vi "mini-proj.vi"() -> ()   [LabVIEW 2013]
uses:
  <vilib>/DAQmx/read.llb/DAQmx Read (Analog 1D Wfm NChan NSamp).vi
  <vilib>/DAQmx/miscellaneous.llb/DAQmx Fill In Error Info.vi
panel:
  out "rpm":dbl
  out "Graphe":waveform(dbl)[](graph)
  in  "Nom de tâche DAQmx":refnum<k21>
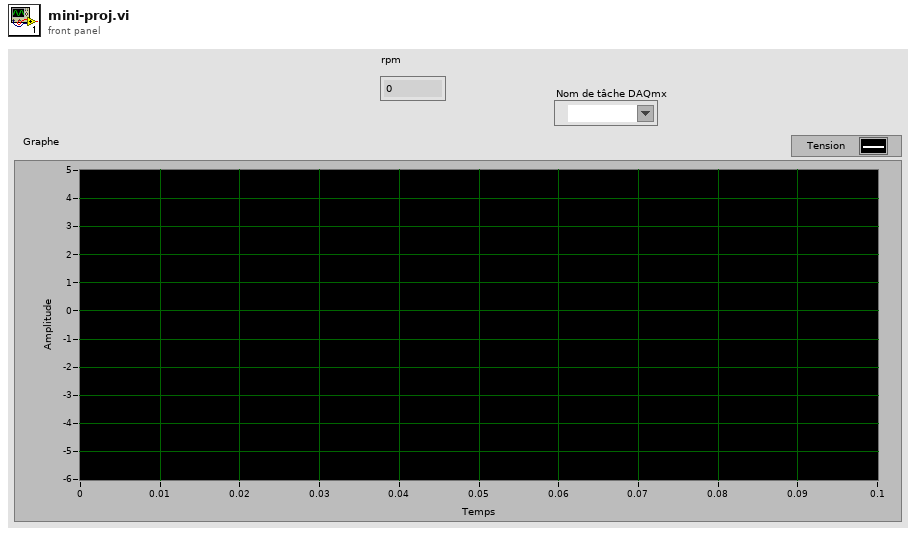
[diagram p1: front panel]
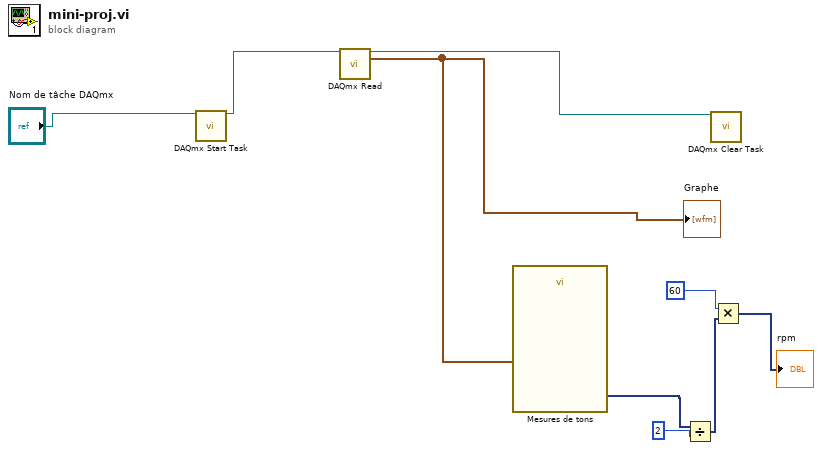
[diagram p0: block diagram]
diagram:
  n1 = call <vilib>:"DAQmx Start Task.vi"("task/channels in"="Nom de tâche DAQmx") -> ("task out"=w7:refnum<k21>)  [unwired: 13 in, 1 out]
  n2 = call-poly <vilib>:"DAQmx Read.vi"("task/channels in"=w7) -> ("task out"=w8:refnum<k21>, "data"=w6:waveform(dbl)[])  [unwired: 12 in, 1 out]
  "Graphe" <- w6
  n3 = call "Mesures de tons"("Signals"=w6) -> ("Frequency"=w5:dynamicdata)  [unwired: 8 in, 2 out]
  n4 = Divide(x=w5, y=2) -> (x/y=w2:dynamicdata)
  n5 = call <vilib>:"DAQmx Clear Task.vi"("task in"=w8) -> ()  [unwired: 14 in, 1 out]
  n6 = Multiply(x=60, y=w2) -> (x*y=→"rpm":dynamicdata)
